vi "Serial Read.vi"(8 "Error In":errorcluster, 10 "Bytes To Read":u32, 11 "LINX Device Config":T1) -> (0 "Error Out":errorcluster, 2 "Data":string, 3 "LINX Device Config":T1)   [LabVIEW 2011, in "LVH-LINX.lvlib"]
doc: "Read data from the serial port associated with the LINX device."
uses:
  LVH-LINX.lvlib
  Type Defs/LINX Device Config.ctl
  Type Defs/Interface.ctl
  Type Defs/TCP Config.ctl
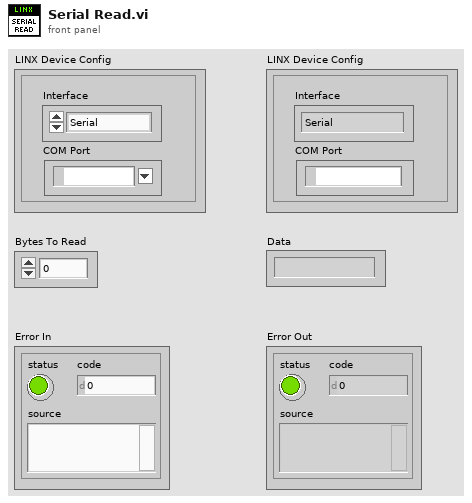
[diagram p1: front panel]
types:
  T1 = typedef "LVH-LINX.lvlib/LINX Device Config.ctl" = cluster{"Interface":T2, "COM Port":refnum<visa-resource-name>, "Packet Number":u16, "TCP Configuration":T3}
  T2 = typedef "LVH-LINX.lvlib/Interface.ctl" = enum16{"Serial", "TCP"}
  T3 = typedef "LVH-LINX.lvlib/TCP Config.ctl" = cluster{"IP Address":string, "Port":dbl}
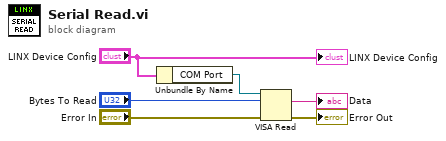
[diagram p0: block diagram]
diagram:
  n1 = Unbundle By Name("LINX Device Config") -> ("COM Port"=w5:refnum<visa-resource-name>)
  n2 = VISA Read(VISA resource name=w5, byte count="Bytes To Read", error in (no error)="Error In") -> (read buffer=→"Data":string, error out=→"Error Out":errorcluster)  [unwired: 2 out]
  "LINX Device Config" <- "LINX Device Config"
